vi "CurrentCellDirtyStateChanged Event Callback.vi"(4 "DataGridView in":refnum<class "DataGridView.lvclass">, 5 "Event Data":cluster{"sender":refnum<k24>, "e":refnum<k24>}, 6 "Control Ref":refnum<k24>, 7 "Event Common Data":T1) -> ()   [LabVIEW 2013, in "DataGrid.lvlib" / "DataGridView.lvclass"]
uses:
  DataGridView/DataGridView.lvclass
  System.Windows.Forms
panel:
  out "CommitEdit":bool
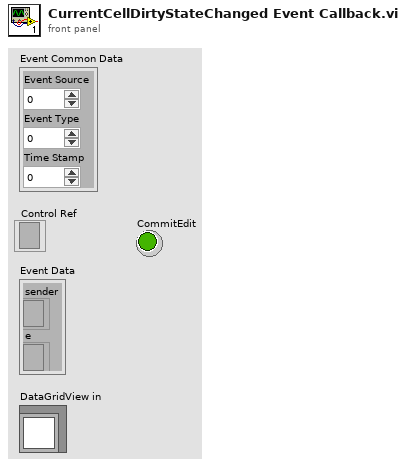
[diagram p1: front panel]
types:
  T1 = cluster{"Event Source":i32, "Event Type":u32, "Time Stamp":u32}
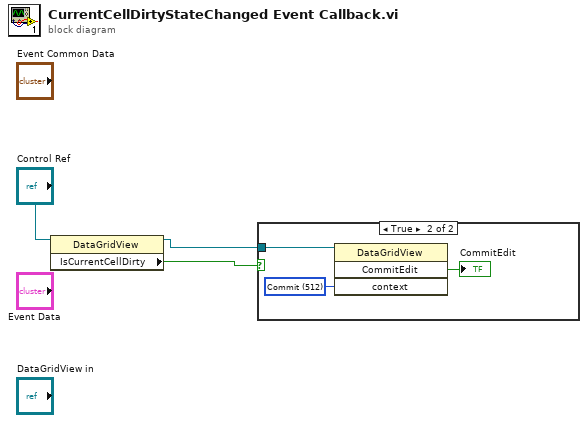
[diagram p0: block diagram]
diagram:
  n1 = property class="DataGridView"(reference="Control Ref") -> (reference out=w3:refnum<k24>, "IsCurrentCellDirty"=w2:bool)  [unwired: 1 in, 1 out]
  n2 = case shown="True" w2 {
    tunnel: w3 -> [_ w6]
    frame False {
    }
    frame True {
      w5 = 512 items=["Formatting"=1, "Display"=2, "PreferredSize"=4, "RowDeletion"=8, "Parsing"=256, "Commit"=512, "InitialValueRestoration"=1024, "LeaveControl"=2048, "CurrentCellChange"=4096, "Scroll"=8192, "ClipboardContent"=16384] ("context")
      n3 = invoke class="DataGridView" method="CommitEdit"(reference=w6, "context"=w5) -> ("CommitEdit"=→"CommitEdit":bool)  [unwired: 2 in, 3 out]
    }
  }
